vi "extract patterns.vi"(8 "end points in":i32[](array[numeric]), 9 "Start points in":i32[](array[numeric]), 11 "player movement data":i32[](array[numeric])) -> (1 "Sub pattern count":i32[](array[numeric]), 2 "Sub patterns":string[](array[string]), 3 "Full movement patterns":string[](array[string]))   [LabVIEW 2013]
panel:
  out "Array 6":i32[](array[numeric])
  out "Array 4":string[](array[string])
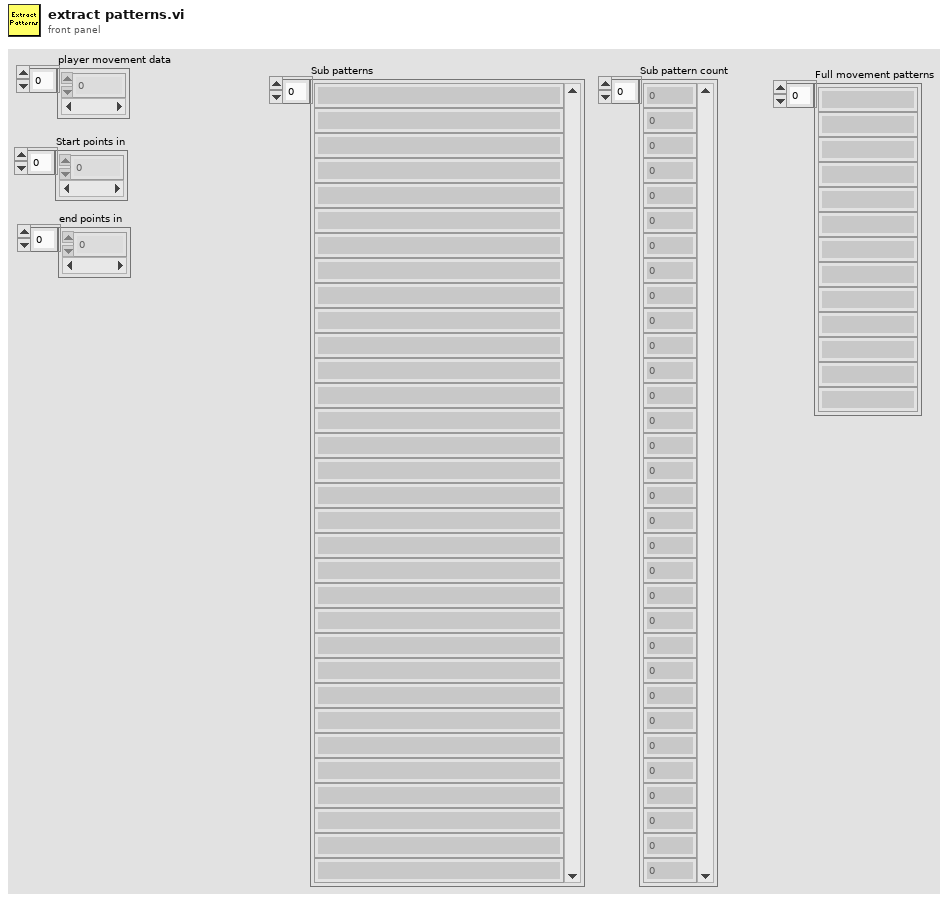
[diagram p1: front panel]
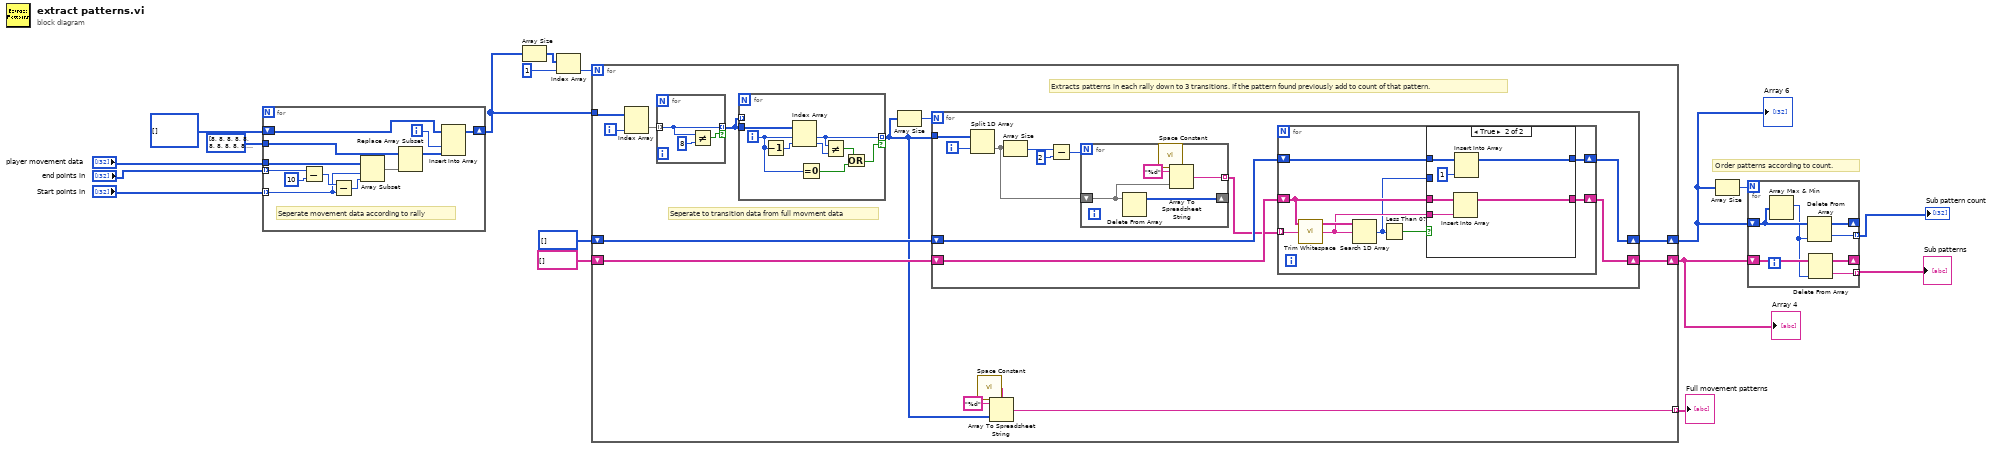
[diagram p0: block diagram]
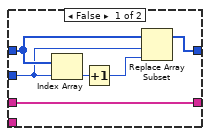
[diagram p2: hidden frame]
diagram:
  # "Order patterns according to count."
  n1 = for {
    tunnel: i32[] [8, 8, 8, 8, 8, 8, 8, 8, 8, 8, 8, 8, 8, 8, 8, 8, 8, 8, 8, 8, 8, 8, 8, 8, 8, 8, 8, 8, 8, 8, 8, 8, 8, 8, 8, 8, 8, 8, 8, 8, 8, 8, 8, 8, 8, 8, 8, 8, 8, 8, 8, 8, 8, 8, 8, 8, 8, 8, 8, 8, 8, 8, 8, 8, 8, 8, 8, 8, 8, 8, 8, 8, 8, 8, 8, 8, 8, 8, 8, 8, 8, 8, 8, 8, 8, 8, 8, 8, 8, 8, 8, 8, 8, 8, 8, 8, 8, 8, 8, 8, 8, 8, 8, 8, 8, 8, 8, 8, 8, 8, 8, 8, 8, 8, 8, 8, 8, 8, 8, 8, 8, 8, 8, 8, 8, 8, 8, 8, 8, 8, 8, 8, 8, 8, 8, 8, 8, 8, 8, 8, 8, 8, 8, 8, 8, 8, 8, 8, 8, 8, 8, 8, 8, 8, 8, 8, 8, 8, 8, 8, 8, 8, 8, 8, 8, 8, 8, 8, 8, 8, 8, 8, 8, 8, 8, 8, 8, 8, 8, 8, 8, 8, 8, 8, 8, 8, 8, 8, 8, 8, 8, 8, 8, 8, 8, 8, 8, 8, 8, 8, 8, 8, 8, 8, 8, 8, 8, 8, 8, 8, 8, 8, 8, 8, 8, 8, 8, 8, 8, 8, 8, 8, 8, 8, 8, 8, 8, 8, 8, 8, 8, 8, 8, 8, 8, 8, 8, 8, 8, 8, 8, 8, 8, 8, 8, 8, 8, 8, 8, 8, 8, 8, 8, 8, 8, 8, 8, 8, 8, 8, 8, 8, 8, 8, 8, 8, 8, 8, 8, 8, 8, 8, 8, 8, 8, 8, 8, 8, 8, 8, 8, 8, 8, 8, 8, 8, 8, 8, 8, 8, 8, 8, 8, 8, 8, 8, 8, 8, 8, 8, 8, 8, 8, 8, 8, 8, 8, 8, 8, 8, 8, 8, 8, 8, 8, 8, 8, 8, 8, 8, 8, 8, 8, 8, 8, 8, 8, 8, 8, 8, 8, 8, 8, 8, 8, 8, 8, 8, 8, 8, 8, 8, 8, 8, 8, 8, 8, 8, 8, 8, 8, 8, 8, 8, 8, 8, 8, 8, 8, 8, 8, 8, 8, 8, 8, 8, 8, 8, 8, 8, 8, 8, 8, 8, 8, 8, 8, 8, 8, 8, 8, 8, 8, 8, 8, 8, 8, 8, 8, 8, 8, 8, 8, 8, 8, 8, 8, 8, 8, 8, 8, 8, 8, 8, 8, 8, 8, 8, 8, 8, 8, 8, 8, 8, 8, 8, 8, 8, 8, 8, 8, 8, 8, 8, 8, 8, 8, 8, 8, 8, 8, 8, 8, 8, 8, 8, 8, 8, 8, 8, 8, 8, 8, 8, 8, 8, 8, 8, 8, 8, 8, 8, 8, 8, 8, 8, 8, 8, 8, 8, 8, 8, 8, 8, 8, 8, 8, 8, 8, 8, 8, 8, 8, 8, 8, 8, 8, 8, 8, 8, 8, 8, 8, 8, 8, 8, 8, 8, 8, 8, 8, 8, 8, 8, 8, 8, 8, 8, 8, 8, 8] -> [w23]
    tunnel: "end points in" -> [w29] mode=indexing
    tunnel: "Start points in" -> [w25] mode=indexing
    tunnel: "player movement data" -> [w26]
    shift-right: [w21] -> w2
    shift-left: i32[][] [] -> [w22]
    i -> [w18]
    # "Seperate movement data according to rally"
    n2 = Subtract(x=w29, y=10) -> (x-y=w27:i32)
    n3 = Subtract(x=w27, y=w25) -> (x-y=w24:i32)
    n4 = Array Subset(array=w26, index=w25, length=w24) -> (w19:i32[])
    n5 = Replace Array Subset(array=w23, new element=w19) -> (w20:i32[])  [unwired: 1 in]
    n6 = Insert Into Array(array=w22, index (col)=w18, new element=w20) -> (w21:i32[][])  [unwired: 1 in]
  }
  n7 = Array Size(array=w2) -> (size(s)=w13:i32[])
  n8 = Index Array(array=w13, index=1) -> (element=w5:i32)
  n9 = for {
    N: w5 -> [_]
    tunnel: w2 -> [w38]
    shift-right: [w41] -> w3
    shift-left: i32[] [] ("Array") -> [w36]
    shift-right: [w42] -> w11
    shift-left: string[] [] -> [w37]
    tunnel: [w30] -> w1 mode=indexing
    i -> [w35]
    # "Extracts patterns in each rally down to 3 transitions. If the pattern found previously add to count of that pattern."
    # "Seperate to transition data from full movment data"
    n10 = Index Array(array=w38, index (col)=w35) -> (element=w40:i32[])  [unwired: 1 in]
    n11 = for {
      tunnel: w40 -> [w53] mode=indexing
      tunnel: [w53] -> w39 mode=indexing if=w51
      n12 = Not Equal?(x=w53, y=8) -> (x != y?=w51:bool)
    }
    n13 = for {
      tunnel: w39 -> [_] mode=indexing
      tunnel: w39 -> [w50]
      tunnel: [w47] -> w31 mode=indexing if=w43
      i -> [w46]
      n14 = Decrement(x=w46) -> (x-1=w49:i32)
      n15 = Index Array(array=w50, index #1=w46, index #2=w49) -> (element #1=w47:i32, element #2=w48:i32)
      n16 = Equal To 0?(x=w46) -> (x = 0?=w44:bool)
      n17 = Not Equal?(x=w47, y=w48) -> (x != y?=w45:bool)
      n18 = Or(x=w45, y=w44) -> (x .or. y?=w43:bool)
    }
    n19 = Array Size(array=w31) -> (size(s)=w34:i32)
    n20 = for {
      N: w34 -> [_]
      tunnel: w31 -> [w57]
      shift-right: [w61] -> w42
      shift-left: w37 -> [w58]
      shift-right: [w60] -> w41
      shift-left: w36 -> [w59]
      i -> [w56]
      n21 = Split 1D Array(array=w57, index=w56) -> (second subarray=w54:i32[])  [unwired: 1 out]
      n22 = Array Size(array=w54) -> (size(s)=w64:i32)
      n23 = Subtract(x=w64, y=2) -> (x-y=w62:i32)
      n24 = for {
        N: w62 -> [_]
        shift-right: [w86] -> _
        shift-left: w54 -> [w85]
        tunnel: [w87] -> w55 mode=indexing
        n25 = Delete From Array(array=w85) -> (array with subset deleted=w86:i32[])  [unwired: 2 in, 1 out]
        n26 = call <vilib>:"Space Constant.vi"() -> ("String"=w89:string)
        n27 = Array To Spreadsheet String(delimiter (Tab)=w89, array=w85, 3:"%d" ("format string")) -> (spreadsheet string=w87:string)
      }
      n28 = for {
        tunnel: w55 -> [w68] mode=indexing
        shift-right: [w71] -> w61
        shift-left: w58 -> [w72]
        shift-right: [w66] -> w60
        shift-left: w59 -> [w67]
        n29 = call <vilib>:"Trim Whitespace.vi"("string"=w68) -> ("trimmed string"=w69:string)  [unwired: 1 in]
        n30 = Search 1D Array(1D array=w72, element=w69) -> (index of element=w65:i32)  [unwired: 1 in]
        n31 = Less Than 0?(x=w65) -> (x < 0?=w70:bool)
        n32 = case shown="True" w70 {
          tunnel: w72 -> [w78 w84]
          tunnel: w69 -> [_ w83]
          tunnel: [w78 w82] -> w71
          tunnel: w67 -> [w76 w81]
          tunnel: [w73 w79] -> w66
          tunnel: w65 -> [w74 _]
          frame False {
            n33 = Index Array(array=w76, index=w74) -> (element=w77:i32)
            n34 = Increment(x=w77) -> (x+1=w75:i32)
            n35 = Replace Array Subset(array=w76, new element=w75, index=w74) -> (w73:i32[])
          }
          frame True {
            n36 = Insert Into Array(array=w84, new element=w83) -> (w82:string[])  [unwired: 1 in]
            n37 = Insert Into Array(array=w81, new element=1 ("new element/subarray")) -> (w79:i32[])  [unwired: 1 in]
          }
        }
      }
    }
    n38 = call <vilib>:"Space Constant.vi"() -> ("String"=w32:string)
    n39 = Array To Spreadsheet String(delimiter (Tab)=w32, array=w31, 3:"%d" ("format string")) -> (spreadsheet string=w30:string)
  }
  "Array 4" <- w11
  "Array 6" <- w3
  "Full movement patterns" <- w1
  n40 = Array Size(array=w3) -> (size(s)=w4:i32)
  n41 = for {
    N: w4 -> [_]
    shift-right: [w95] -> _
    shift-left: w3 -> [w96]
    tunnel: [w94] -> w9 mode=indexing
    shift-right: [w91] -> _
    shift-left: w11 -> [w93]
    tunnel: [w90] -> w10 mode=indexing
    n42 = Array Max & Min(array=w96) -> (max index (indices)=w92:i32)  [unwired: 3 out]
    n43 = Delete From Array(array=w96, index=w92) -> (deleted portion=w94:i32, array with subset deleted=w95:i32[])  [unwired: 1 in]
    n44 = Delete From Array(array=w93, index=w92) -> (deleted portion=w90:string, array with subset deleted=w91:string[])  [unwired: 1 in]
  }
  "Sub pattern count" <- w9
  "Sub patterns" <- w10
